vi "ReadScores.vi"(8 "error in (no error)":errorcluster, 11 "Controller in":refnum<class "Controller.lvclass">) -> (0 "error out":errorcluster, 2 "Scores":string[][](table) caption="Result Set (from first statement with results)", 3 "Controller out":refnum<class "Controller.lvclass">)   [LabVIEW 2024, in "GUI.lvlib" / "Controller.lvclass"]
uses:
  Controller.lvclass
  Controller.lvclass/Controller.ctl
  <vilib>/drjdpowell/SQLite Library/SQLite.lvlib
  <vilib>/drjdpowell/SQLite Library/SQL Connection/Execute SQL.vi
  <vilib>/drjdpowell/SQLite Library/SQL Connection/Connection.lvclass
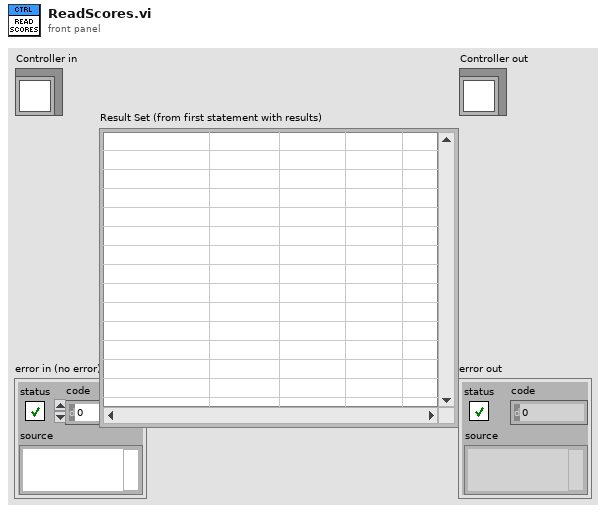
[diagram p1: front panel]
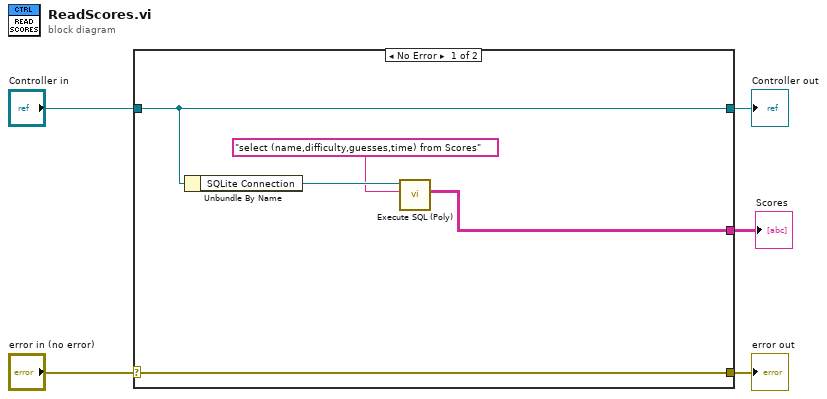
[diagram p0: block diagram]
diagram:
  n1 = case shown="No Error" "error in (no error)" {
    selector: "error in (no error)" -> [w10 w12]
    tunnel: [w10 w12] -> w4
    tunnel: [w7 w11] -> w2
    tunnel: "Controller in" -> [w7 w11]
    tunnel: [w6 _] -> w1
    frame No Error {
      n2 = Unbundle By Name(w7) -> ("SQLite Connection"=w9:refnum<class "Connection.lvclass">)
      n3 = call-poly <vilib>:"Execute SQL (Poly).vi"("SQL"="select (name,difficulty,guesses,time) from Scores", "SQLite Connection in"=w9) -> ("Result Set"=w6:string[][])  [unwired: 6 in, 3 out]
    }
    frame Error {
    }
  }
  "error out" <- w4
  "Controller out" <- w2
  "Scores" <- w1
